vi "Add New Mock to Project.vi"(8 "error in (no error)":errorcluster, 11 "Mock Class Generator in":refnum<class "Mock Class Generator.lvclass">) -> (0 "error out":errorcluster, 3 "Mock Class Generator out":refnum<class "Mock Class Generator.lvclass">)   [LabVIEW 2020, in "Mock Class Generator.lvclass"]
uses:
  Mock Class Generator.lvclass
  Mock Class Generator.lvclass/Mock Class Generator.ctl
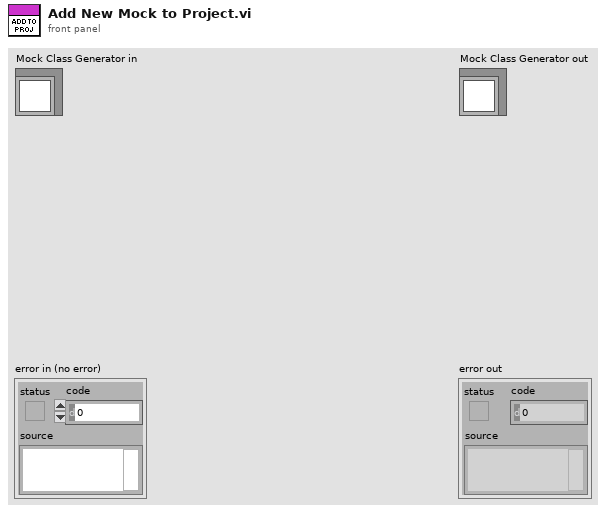
[diagram p1: front panel]
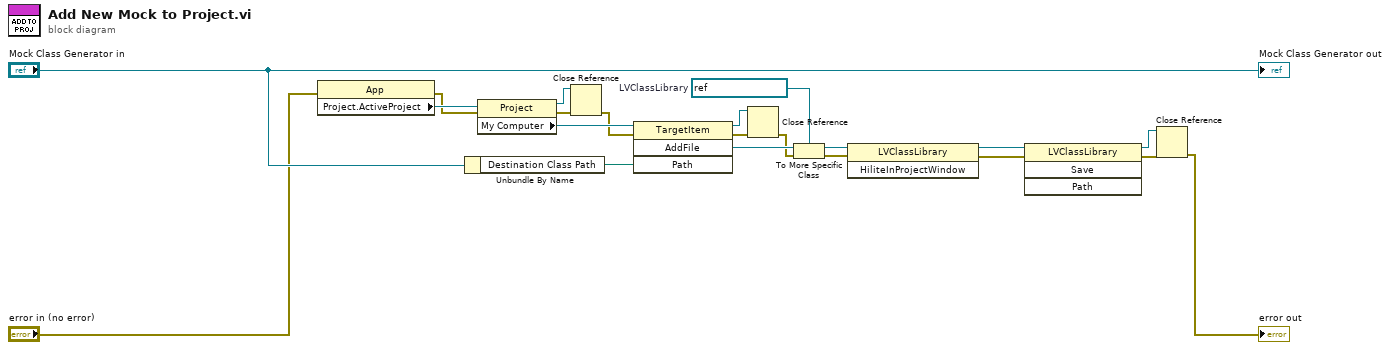
[diagram p0: block diagram]
diagram:
  w13 = refnum<vi> refnum  # LVClassLibrary
  n1 = property class="App"(error in="error in (no error)") -> (error out=w12:errorcluster, "Project.ActiveProject"=w17:refnum<vi>)  [unwired: 1 in, 1 out]
  n2 = Unbundle By Name("Mock Class Generator in") -> ("Destination Class Path"=w15:path)
  n3 = property class="Project"(reference=w17, error in=w12) -> (reference out=w10:refnum<vi>, error out=w11:errorcluster, "My Computer"=w16:refnum<vi>)
  n4 = Close Reference(reference=w10, error in (no error)=w11) -> (error out=w9:errorcluster)
  n5 = invoke class="TargetItem" method="AddFile"(reference=w16, error in=w9, "Path"=w15) -> (reference out=w8:refnum<vi>, error out=w7:errorcluster, "AddFile"=w14:refnum<vi>)  [unwired: 1 in, 1 out]
  n6 = Close Reference(reference=w8, error in (no error)=w7) -> (error out=w6:errorcluster)
  n7 = To More Specific Class(target class=w13, reference=w14, error in=w6) -> (specific class reference=w4:refnum<vi>, error out=w2:errorcluster)
  n8 = invoke class="LVClassLibrary" method="HiliteInProjectWindow"(reference=w4, error in=w2) -> (reference out=w3:refnum<vi>, error out=w1:errorcluster)  [unwired: 1 in, 1 out]
  n9 = invoke class="LVClassLibrary" method="Save"(reference=w3, error in=w1) -> (reference out=w18:refnum<vi>, error out=w19:errorcluster)  [unwired: 2 in, 2 out]
  n10 = Close Reference(reference=w18, error in (no error)=w19) -> (error out=→"error out":errorcluster)
  "Mock Class Generator out" <- "Mock Class Generator in"
